vi "Add float (multiple).vi"(8 "error in (no error)":errorcluster, 10 "y":dbl, 11 "Multiple XY-data in":cluster{"X-array":dbl[], "Y-array":dbl[]}[](array[cluster]) {"Y-array" format="%.2p"; "X-array" format="%.2p"}) -> (0 "error out":errorcluster, 3 "Multiple XY-data out":cluster{"X-array":dbl[], "Y-array":dbl[]}[](array[cluster]) {"Y-array" format="%.2p"; "X-array" format="%.2p"})   [LabVIEW 2016, in "xy_utilities.lvlib"]
uses:
  xy_utilities.lvlib
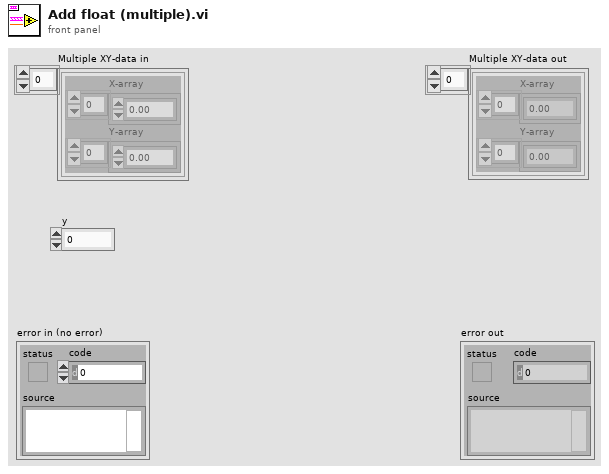
[diagram p1: front panel]
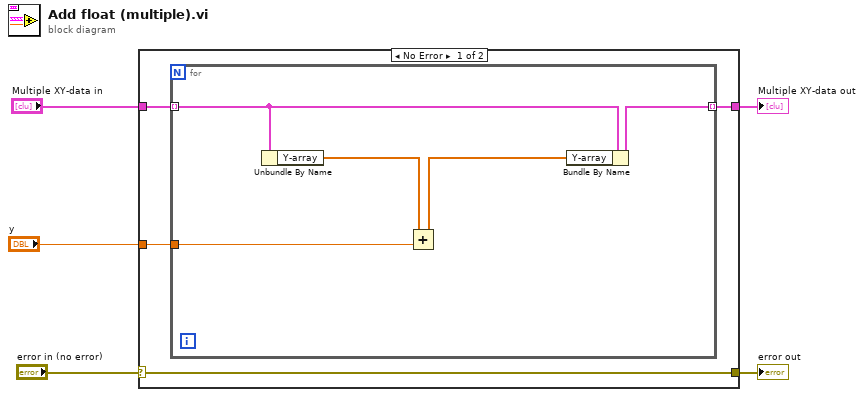
[diagram p0: block diagram]
diagram:
  n1 = case shown="No Error" "error in (no error)" {
    selector: "error in (no error)" -> [w9 w16]
    tunnel: [w9 w16] -> w4
    tunnel: "Multiple XY-data in" -> [w8 w15]
    tunnel: [w7 w15] -> w2
    tunnel: "y" -> [w6 _]
    frame No Error {
      n2 = for {
        tunnel: w8 -> [w14] mode=indexing
        tunnel: [w13] -> w7 mode=indexing
        tunnel: w6 -> [w12]
        n3 = Unbundle By Name(w14) -> ("Y-array"=w11:dbl[])
        n4 = Add(x=w11, y=w12) -> (x+y=w10:dbl[])
        n5 = Bundle By Name(cluster=w14, "Y-array"=w10) -> (w13:cluster{"X-array":dbl[], "Y-array":dbl[]})
      }
    }
    frame Error {
    }
  }
  "error out" <- w4
  "Multiple XY-data out" <- w2
